vi "Add Property (Enum).vi"(7 "Required?":bool, 8 "error in (no error)":errorcluster, 9 "Enum In":refnum<vi>, 11 "JSON Schema in":string) -> (0 "error out":errorcluster, 3 "JSON SChema out":string)   [LabVIEW 2020, in "JSON Schema Generator.lvlib"]
uses:
  JSON Schema Generator.lvlib
  298c09ea-0ead-4ea4-aadc-fafb17d6c281.vi
  <vilib>/JDP Science/JSONtext/Variant to JSON Text.vi
  <vilib>/JDP Science/JSONtext/LVClass Serializer/JSONtext LVClass Serializer.lvclass
  <vilib>/JDP Science/JSONtext/JSONtext.lvlib
  <vilib>/Utility/Data Type/NI_Data Type.lvlib
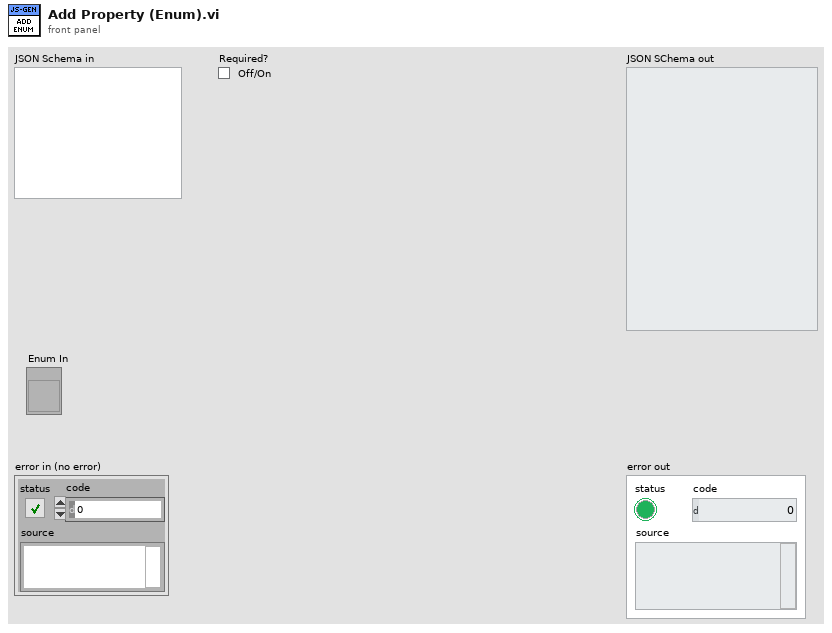
[diagram p1: front panel]
types:
  T1 = typedef "NI_Data Type.lvlib/Data Type.ctl" = enum8{"Invalid Type", "Void", "I8", "I16", "I32", "I64", "U8", "U16", "U32", "U64", "Single Float", "Double Float", "Extended Float", "Single Complex", "Double Complex", "Extended Complex", "Enum U8", "Enum U16", "Enum U32", "Enum U64", "Single Float With Unit", "Double Float With Unit", "Extended Float With Unit", "Single Complex with Unit", "Double Complex with Unit", "Extended Complex with Unit", "Boolean", "String", "Path", "Picture", "Tag", "Array", "Cluster", "Variant", "LV Variant", "Waveform", "Timestamp", "Digital Waveform", "Digital Data", "ExpressData", "Refnum", "External Data", "VI", "Poly VI", "LabVIEW Class Instance", "Fixed Point", "Set Collection", "Map Collection"}
  T2 = typedef "NI_Data Type.lvlib/Type Definition Info.ctl" = cluster{"Name":string, "Timestamp":u32}
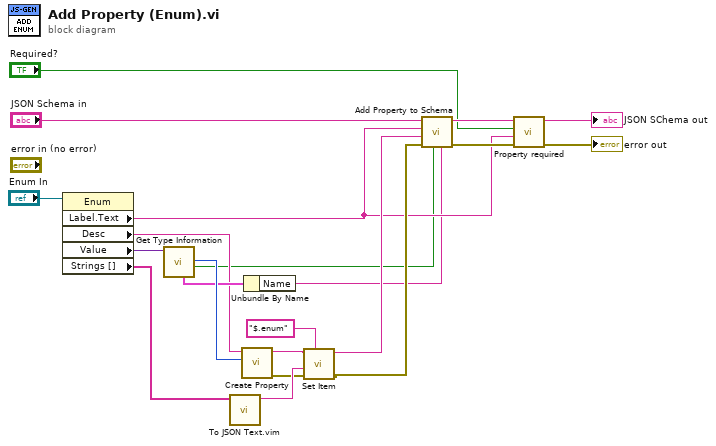
[diagram p0: block diagram]
diagram:
  n1 = property class="Enum"(reference="Enum In") -> ("Label.Text"=w5:string, "Desc"=w3:string, "Value"=w7:variant, "Strings []"=w8:string[])  [unwired: 1 in, 2 out]
  n2 = call <vilib>:"Get Type Information.vi"("variant"=w7) -> ("type definition"=w1:bool, "type"=w6:T1, "type definition info"=w4:T2)  [unwired: 6 in, 2 out]
  n3 = call "To JSON Text.vim"("Anything"=w8) -> ("<JSON>"=w11:string)  [unwired: 9 in, 1 out]
  n4 = call "Create Property.vi"("Labview Type"=w6, "Description"=w3) -> ("error out"=w10:errorcluster, "JSON Schema Property out"=w15:string)  [unwired: 8 in]
  n5 = Unbundle By Name(w4) -> ("Name"=w2:string)
  n6 = call <vilib>:"Set Item.vi"("$Path or Item Name"="$.enum", "error in (no error)"=w10, "JSON to Insert"=w11, "JSON"=w15) -> ("error out"=w14:errorcluster, "<JSON>"=w13:string)  [unwired: 4 in, 1 out]
  n7 = call "Add Property to Schema.vi"("Typedef Name"=w2, "Typedef?"=w1, "error in"=w14, "JSON Schema Property in"=w13, "Property Name"=w5, "JSON Schema in"="JSON Schema in") -> ("error out"=w18:errorcluster, "JSON Schema out"=w21:string)  [unwired: 4 in]
  n8 = call "Property required.vi"("error in (no error)"=w18, "Name"=w5, "Required?"="Required?", "JSON Schema in"=w21) -> ("error out"=→"error out":errorcluster, "JSON Schema out"=→"JSON SChema out":string)  [unwired: 6 in]
